vi "tsapp_clear_can_receive_buffers_win32.vi"(8 "错误输入（无错误）":errorcluster, 10 "AAppChannel":u8) -> (0 "错误输出":errorcluster, 2 "tsapp_clear_can_receive_buffers":i32)   [LabVIEW 2016]
uses:
  TSMaster.dll
panel:
  # "用于清除指定通道的接收缓冲区中的数据"
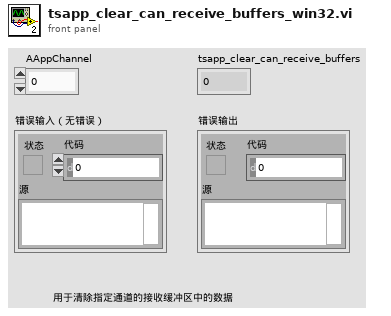
[diagram p1: front panel]
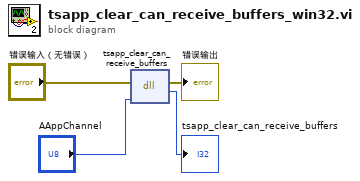
[diagram p0: block diagram]
diagram:
  n1 = dll-call lib="C:/Users/Eric/Desktop/TSCAN_LV2010/TSMaster.dll" fn="tsapp_clear_can_receive_buffers"(error in="错误输入（无错误）", "AChn"="AAppChannel") -> (error out=→"错误输出":errorcluster, "tsapp_clear_can_receive_buffers"=→"tsapp_clear_can_receive_buffers":i32)  [unwired: 3 in, 1 out]
